vi "GageMultipleRecord_mod_seg.vi"() -> ()   [LabVIEW 2017]
uses:
  <instrlib>/niHWS/nihws.llb/niHWS Open File Permissions ID.ctl
  <instrlib>/niHWS/nihws.llb/niHWS Set Wfm DBL Attribute ID.ctl
  <instrlib>/niHWS/nihws.llb/niHWS Set Wfm DBL Attribute.vi
  <instrlib>/niHWS/nihws.llb/niHWS Write Analog I16.vi
panel:
  out "Numeric":i32
  in  "Number Of Records 2":u32=100
  in  "Save HWS to:":path=path "C:/Users/plasma/Desktop/test.hws"
  out "Segment":u32=1 max=10000
  out "Board":string
  in  "Number Of Records":u32=100
  out "1st segment TS":string
  out "Time Interval Graph":cluster{i32[], dbl[]}(graph)
  out "Tick Frequency, Hz":u32
  in  "Run":bool=TRUE
  in  "Trigger":T1={"Slope"=0, "Level"=0, "Source"=0, "External Range"=2000, "External Coupling"=0, "External"=FALSE, "Disable"=FALSE, "External Impedance"=1} {"External Impedance" items=["50 Ohm", "HiZ"]; "External Coupling" items=["DC", "AC"]; "External Range" min=2000 max=10000 step=8000; "Slope" items=["Rising", "Falling"]; "Level" min=-100 max=100; "Source" min=0 max=64 step=1}
  in  "Reset":bool
  in  "Counter source":bool
  out "Array":dbl[](array[numeric]) format="%.2f"
  out "Status":string
  in  "Channels":T2(array[cluster])=[{"Coupling"=0, "Differential Input"=FALSE, "Direct-to-ADC"=FALSE, "Range"=2000, "Impedance"=50, "DC Offset"=0, "Filter"=0}] {"Impedance" min=50 max=1000000 step=999950; "Coupling" items=["DC", "AC"]}
  in  "Acquisition":T3={"Sample Rate"=10000000.0, "Mode"=0, "Depth"=8160.0, "Segment Size"=8160.0, "Trigger Timeout"=1000000.0, "Trigger Holdoff"=0.0, "Trigger Delay"=0.0, "Clock mode"=enum."Internal"} {"Segment Size" min=32.0 step=16.0; "Trigger Delay" min=0.0 step=1.0; "Trigger Holdoff" min=0.0 step=16.0; "Depth" min=0.0 step=16.0; "Mode" items=["Single", "Dual", "Quad", "Octal"]}
  in  "Stop":bool
  in  "Length":dbl=512.0 min=0.0 step=1.0
  in  "Start Point":dbl step=16.0
  out "Waveform Graph":T4(graph) caption="Record 10000  of  10000"
  # "Time stamp"
  # "of"
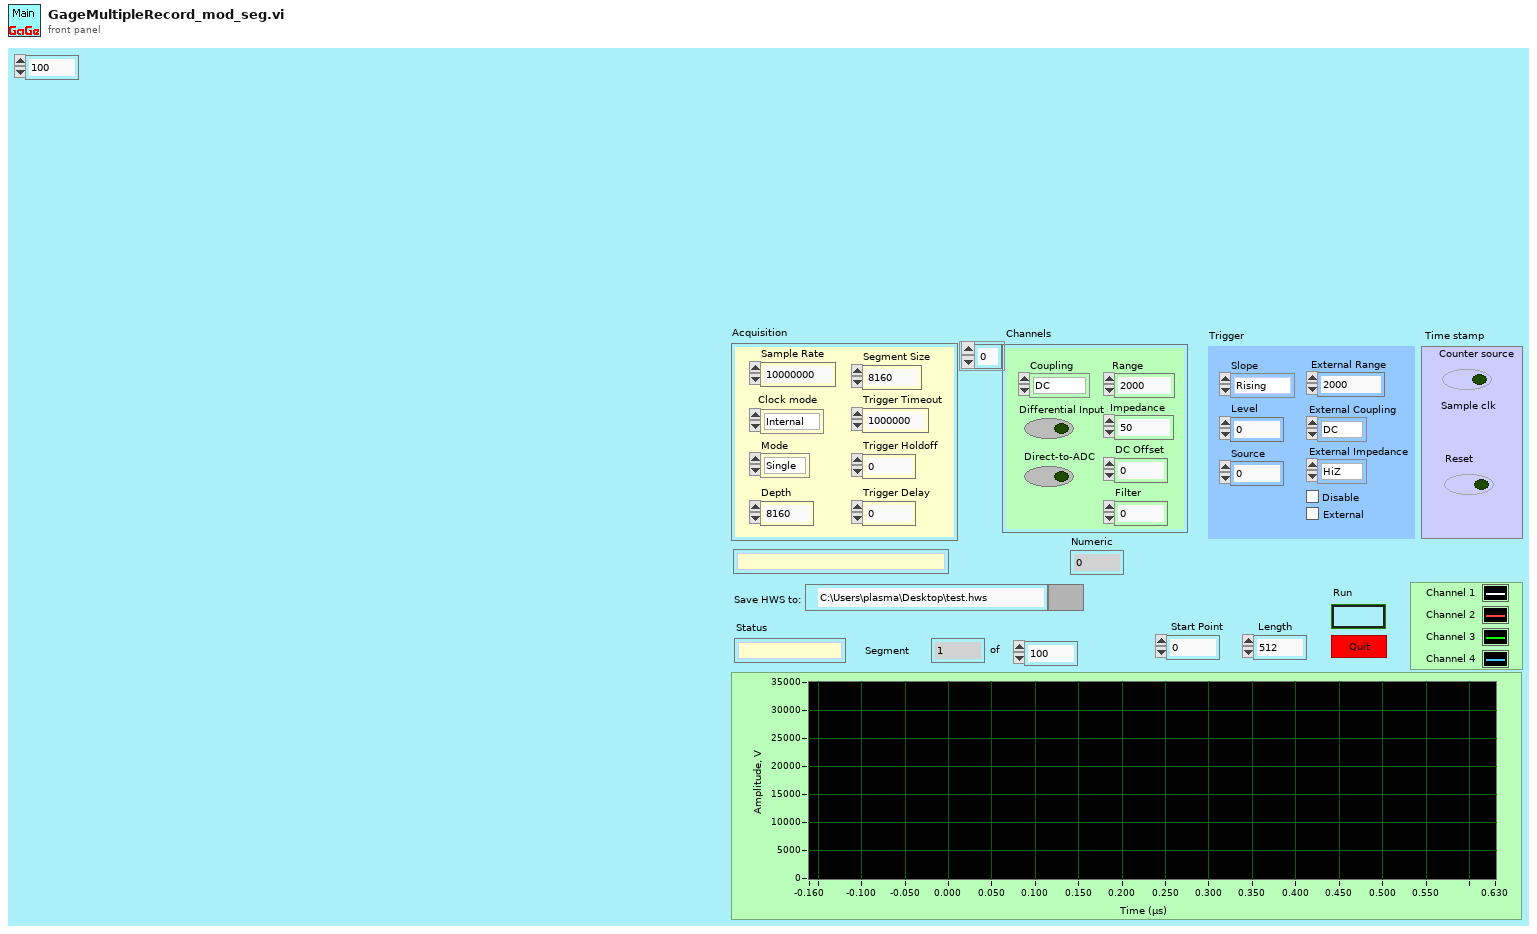
[diagram p1: front panel]
types:
  T1 = cluster{"Slope":u16, "Level":i32, "Source":i32, "External Range":u32, "External Coupling":u16, "External":bool, "Disable":bool, "External Impedance":u16}
  T2 = cluster{"Coupling":u16, "Differential Input":bool, "Direct-to-ADC":bool, "Range":u32, "Impedance":u32, "DC Offset":i32, "Filter":i32}[]
  T3 = cluster{"Sample Rate":dbl, "Mode":u16, "Depth":dbl, "Segment Size":dbl, "Trigger Timeout":dbl, "Trigger Holdoff":dbl, "Trigger Delay":dbl, "Clock mode":enum16{"Internal", "External", "Reference"}}
  T4 = cluster{dbl, dbl, "Data before\n conversion":i16[]}
  T5 = typedef "niHWS Open File Permissions ID.ctl" = enum32{"Read Only", "Read/Write Existing", "Read/Write/Create New", "Read/Write/Create New Always"}
  T6 = cluster{"Handle":u32, "Sample size":u32, "Resolution":i32, "Offset":i32, "Channels":u32, "Boards":u32}
  T7 = cluster{"Coupling":u16, "Differential Input":bool, "Direct-to-ADC":bool, "Range":u32, "Impedance":u32, "DC Offset":i32, "Filter":i32}
  T8 = cluster{string, "Differential Input":bool, "Direct-to-ADC":bool, "Range":u32, "Impedance":u32, "DC Offset":i32, u32}
  T9 = cluster{"RingText.Text":string, "Level":i32, "Source":i32, "External Range":u32, "RingText.Text":string, "External":bool, "Disable":bool, "RingText.Text":string}
  T10 = cluster{"RingText.Text":string, "Level":i32, "Source":i32, "External Range":u32, "RingText.Text":string, "External":bool, "Disable":bool, "RingText.Text":string}[]
  T11 = cluster{"Sample Rate":dbl, "Clock mode":enum16{"Internal", "External", "Reference"}, "RingText.Text":string, "Depth":dbl, "Segment Size":dbl, "Trigger Timeout":dbl, "Trigger Holdoff":dbl, "Trigger Delay":dbl}
  T12 = cluster{"Handle":u32, "Sample Size":u32, "Resolution":i32, "Offset":i32, "Channels":u32, "Boards":u32}
  T13 = typedef "niHWS Set Wfm DBL Attribute ID.ctl" = u32
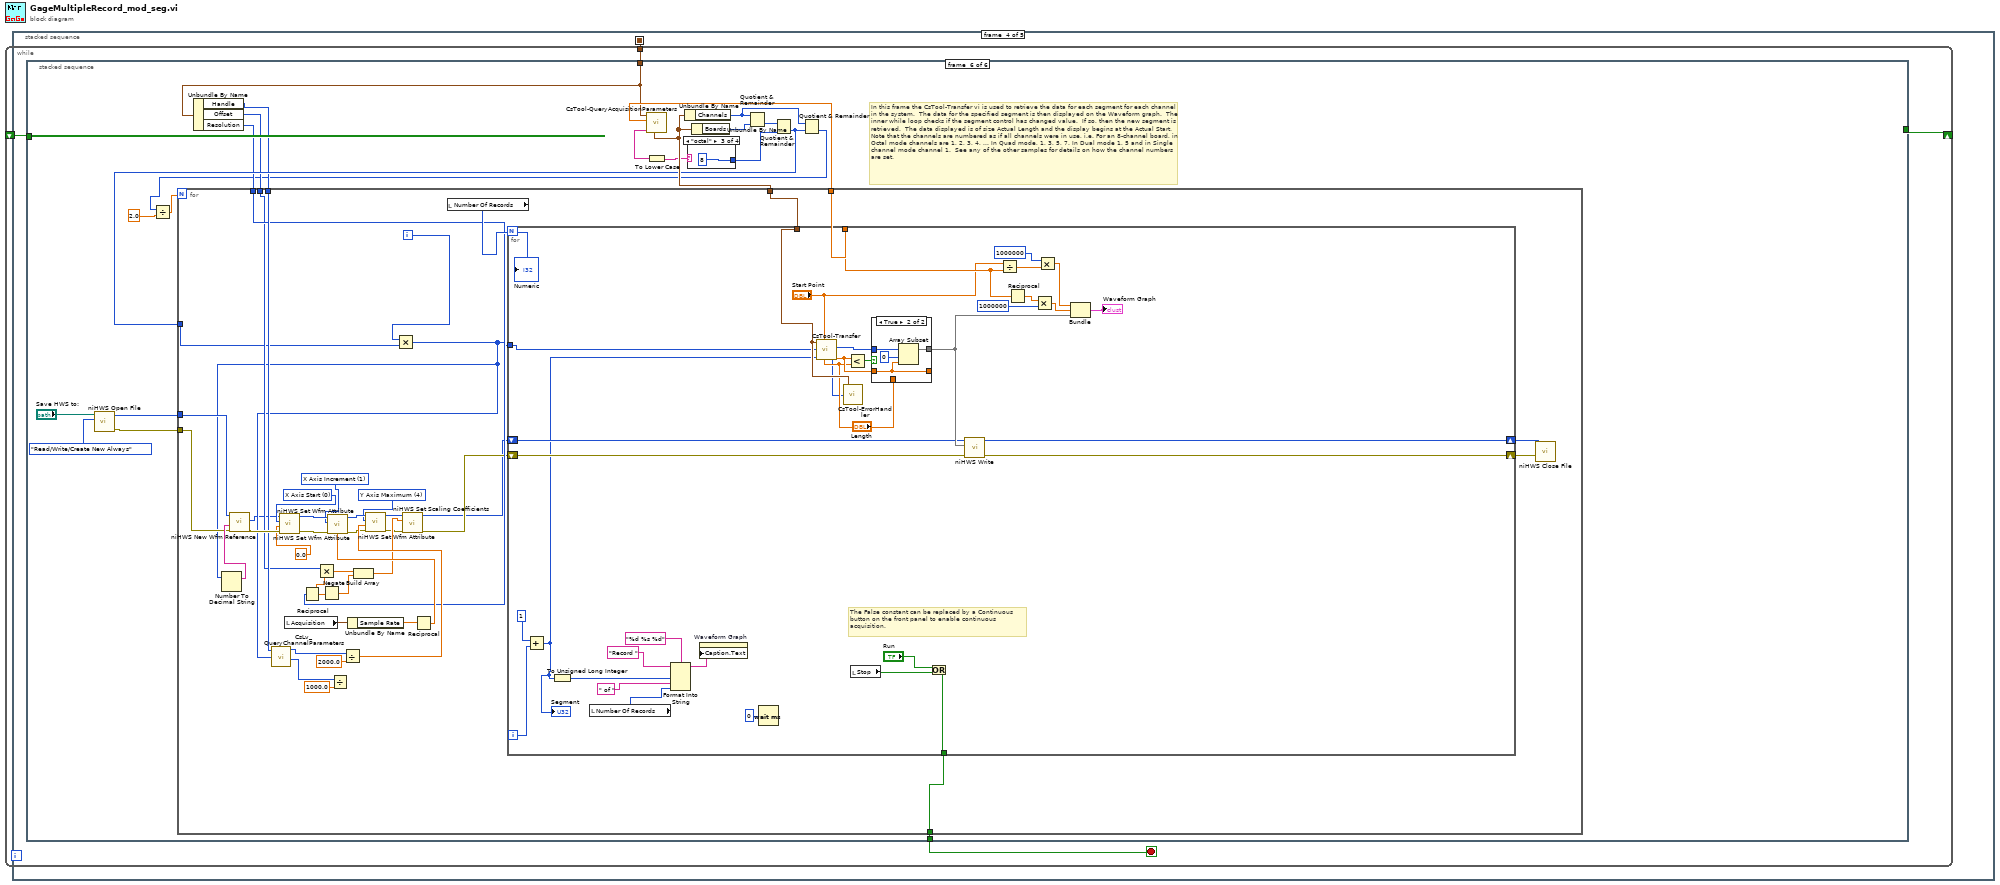
[diagram p0: block diagram]
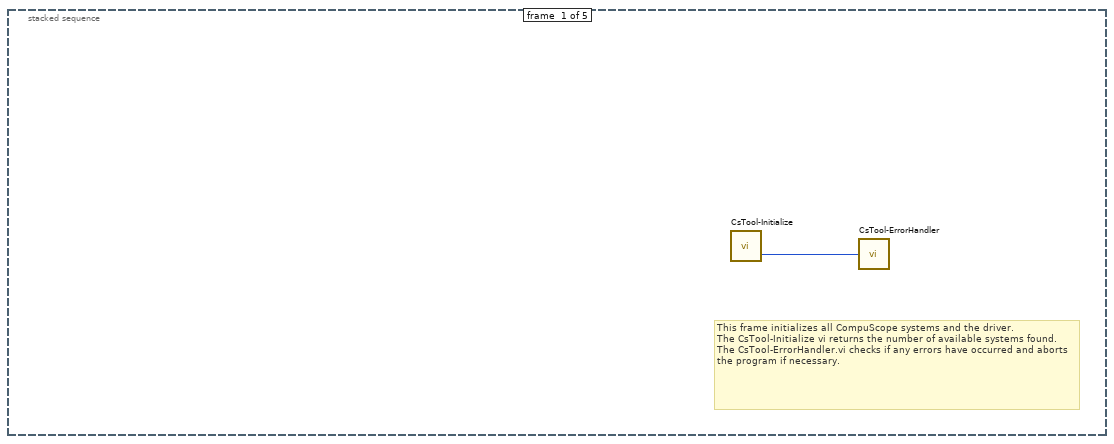
[diagram p2: hidden frame]
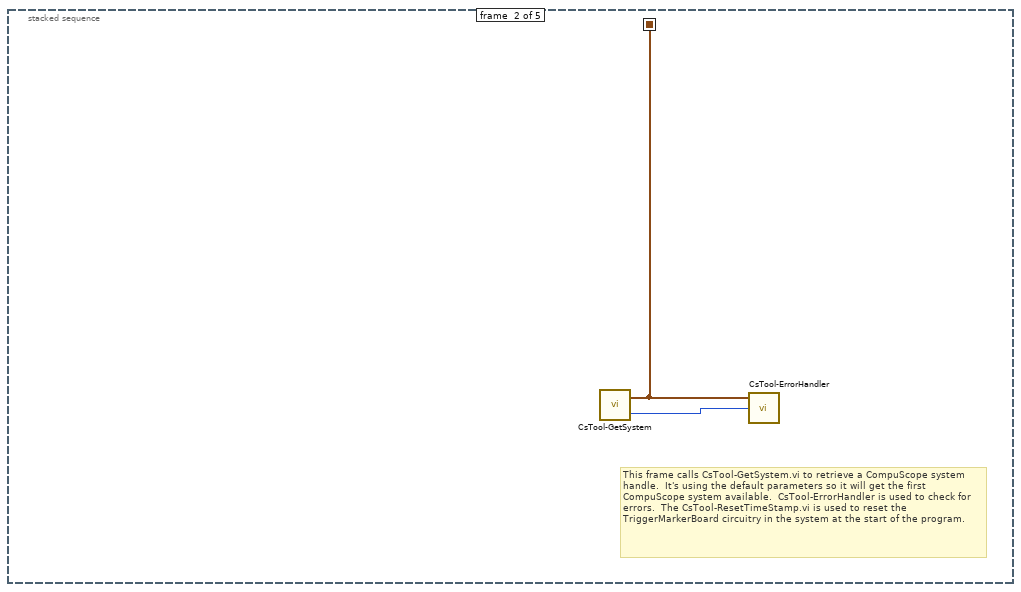
[diagram p3: hidden frame]
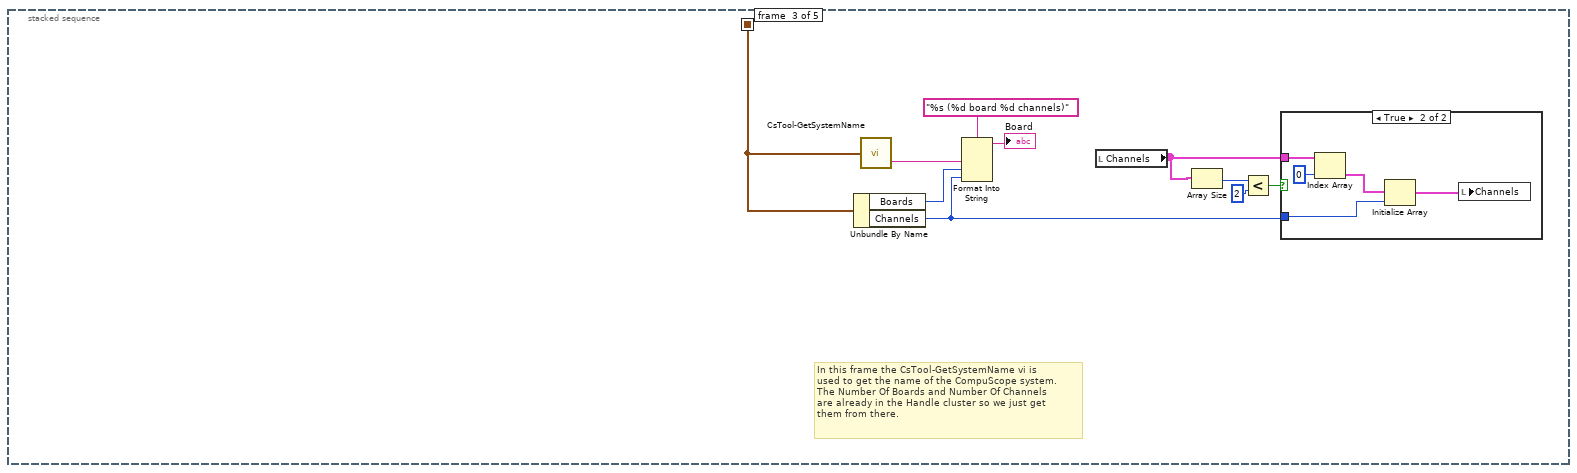
[diagram p4: hidden frame]
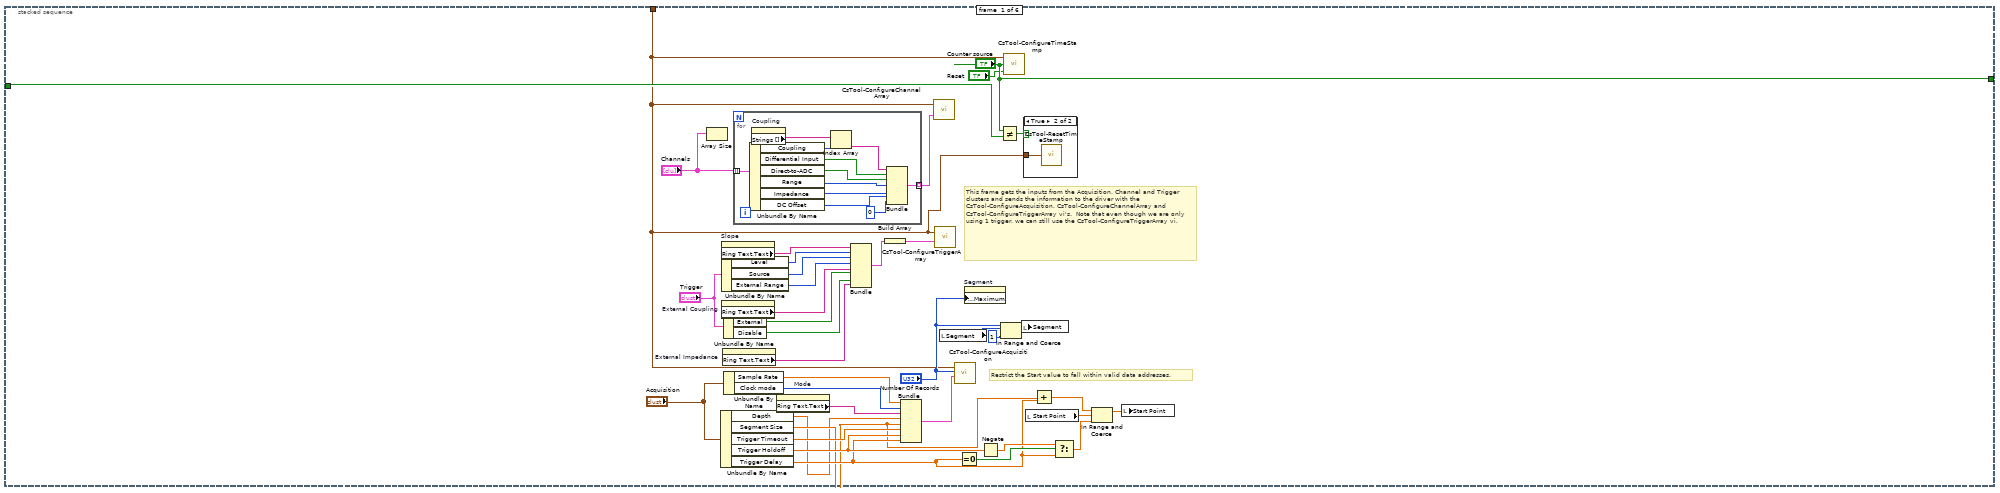
[diagram p6: hidden frame]
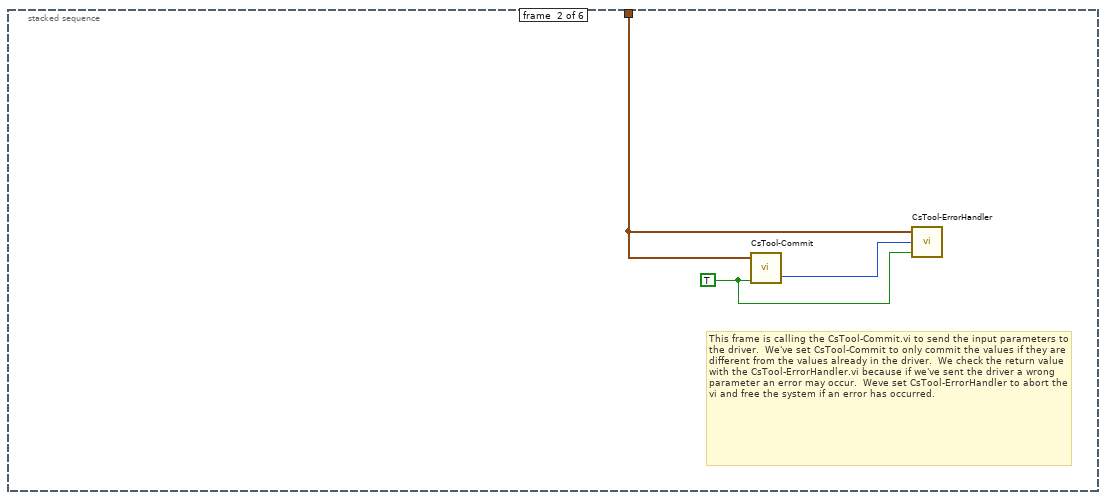
[diagram p8: hidden frame]
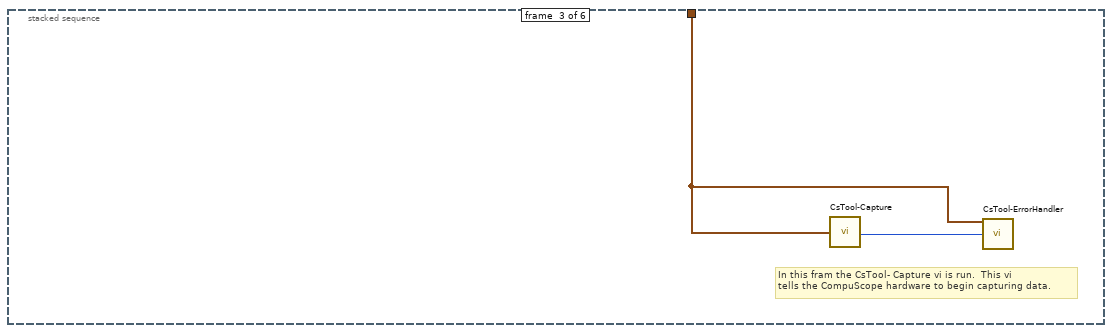
[diagram p9: hidden frame]
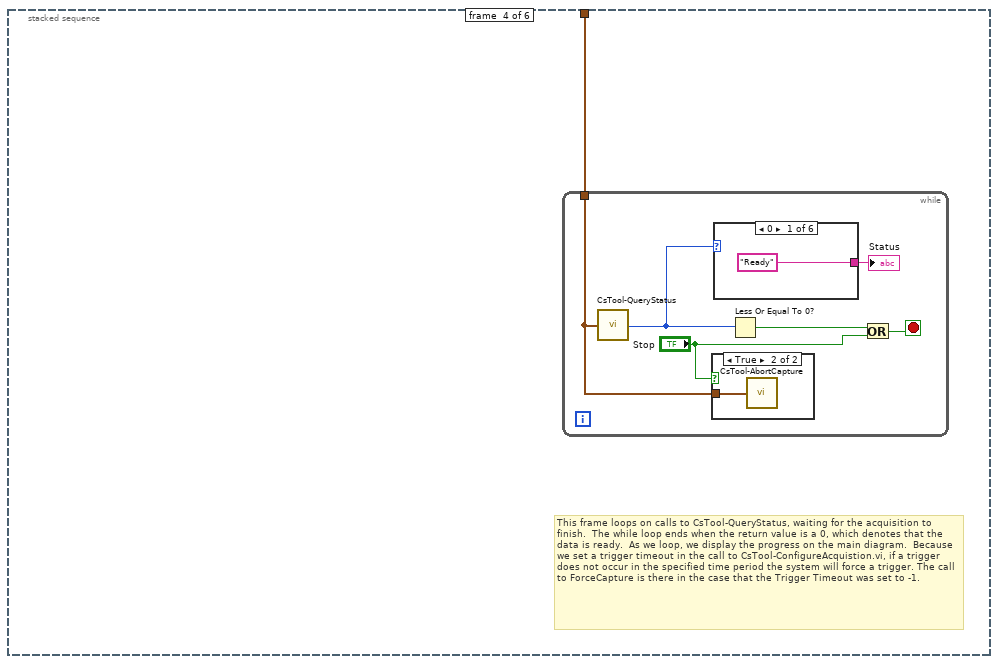
[diagram p10: hidden frame]
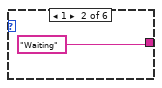
[diagram p12: hidden frame]
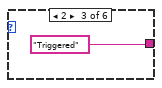
[diagram p13: hidden frame]
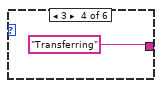
[diagram p14: hidden frame]
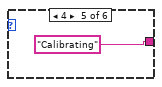
[diagram p15: hidden frame]
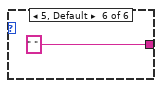
[diagram p16: hidden frame]
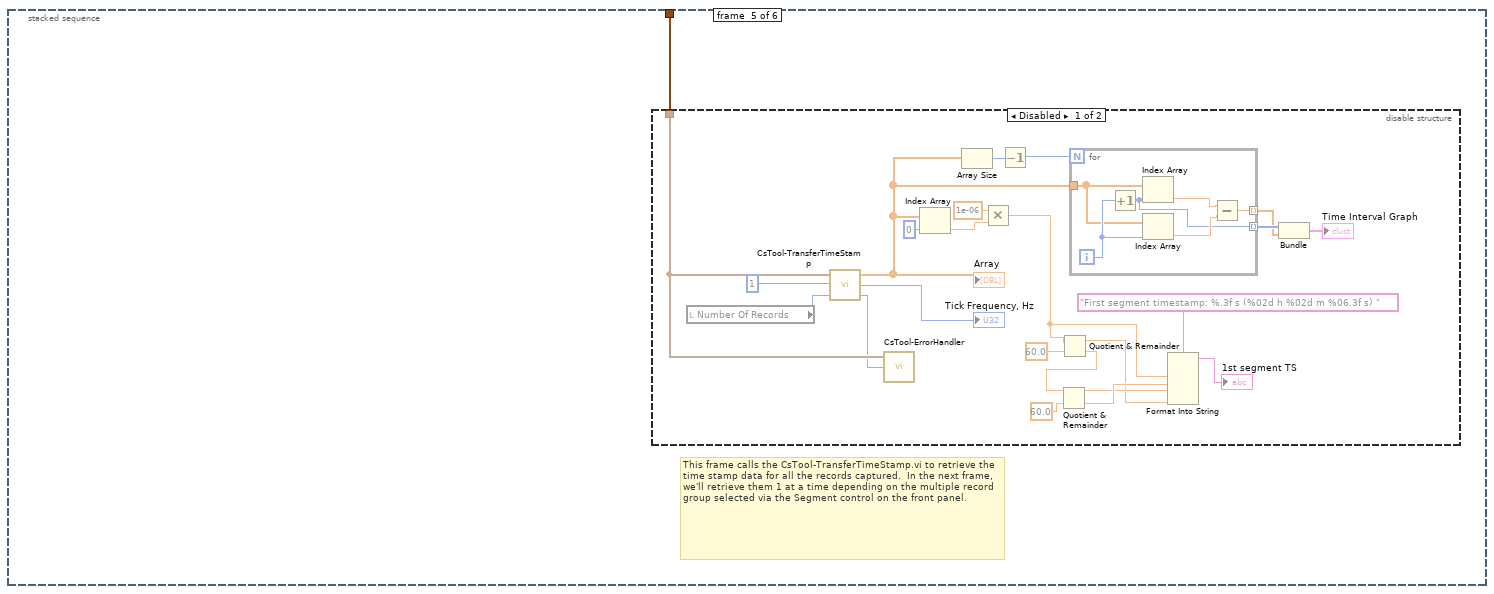
[diagram p17: hidden frame]
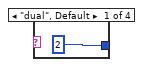
[diagram p20: hidden frame]
diagram:
  n1 = stacked-sequence {
    seq-local: [_ w2 _ _ _] -> [_ _ w13 w19 w231]
    frame #0 {
      # "This frame initializes all CompuScope systems and the driver.\nThe CsTool-Initialize vi returns the number of available systems found.  The CsTool-ErrorHandler.vi checks if any errors have occurred and aborts the program if necessary."
      n2 = call <userlib>:"CsTool-Initialize.vi"() -> ("Error Code"=w1:i32)  [unwired: 1 out]
      n3 = call <userlib>:"CsTool-ErrorHandler.vi"("Error Code"=w1) -> ()  [unwired: 2 in, 1 out]
    }
    frame #1 {
      # "This frame calls CsTool-GetSystem.vi to retrieve a CompuScope system handle.  It's using the default parameters so it will get the first CompuScope system available.  CsTool-ErrorHandler is used to check for errors.  The CsTool-ResetTimeStamp.vi is used to reset the TriggerMarkerBoard circuitry in the system at the start of the program."
      n4 = call <userlib>:"CsTool-GetSystem.vi"() -> ("Error Code"=w3:i32, "Handle Cluster"=w2:T6)  [unwired: 4 in]
      n5 = call <userlib>:"CsTool-ErrorHandler.vi"("Error Code"=w3, "Handle Cluster"=w2) -> ()  [unwired: 1 in, 1 out]
    }
    frame #2 {
      # "In this frame the CsTool-GetSystemName vi is \nused to get the name of the CompuScope system.\nThe Number Of Boards and Number Of Channels \nare already in the Handle cluster so we just get \nthem from there."
      n6 = Unbundle By Name(w13) -> ("Boards"=w5:u32, "Channels"=w6:u32)
      n7 = call <userlib>:"CsTool-GetSystemName.vi"("Handle Cluster"=w13) -> ("System Name"=w7:string)  [unwired: 1 out]
      n8 = Format Into String(format string="%s (%d board %d channels)", w7, w5, w6) -> (resulting string=→"Board":string)  [unwired: 2 in, 1 out]
      n9 = local read "Channels"() -> (w11:T2)
      n10 = Array Size(array=w11) -> (size(s)=w10:i32)
      n11 = Less?(x=w10, y=2) -> (x < y?=w12:bool)
      n12 = case shown="True" w12 {
        tunnel: w6 -> [_ w18]
        tunnel: w11 -> [_ w16]
        frame False {
        }
        frame True {
          n13 = Index Array(array=w16, index=0) -> (element=w15:T7)
          n14 = Initialize Array(w15, w18) -> (w14:T2)
          n15 = local write "Channels"(w14) -> ()
        }
      }
    }
    frame #3 {
      n16 = while {
        tunnel: w19 -> [w23]
        shift-right: [w22] -> _
        shift-left: _ -> [w21]
        stop <- w20 stop-if-true
        n17 = stacked-sequence {
          tunnel: w23 -> [w34 w74 w77 w79 w93 w132]
          tunnel: ["Counter source" _ _ _ _ _] -> w22
          tunnel: w21 -> [w37 _ _ _ _ _]
          tunnel: [_ _ _ _ _ w128] -> w20
          frame #0 {
            # "Restrict the Start value to fall within valid data addresses."
            # "This frame gets the inputs from the Acquisition, Channel and Trigger clusters and sends the information to the driver with the CsTool-ConfigureAcquisition, CsTool-ConfigureChannelArray and CsTool-ConfigureTriggerArray vi's.  Note that even though we are only using 1 trigger, we can still use the CsTool-ConfigureTriggerArray vi."
            n18 = Array Size(array="Channels") -> ()  [unwired: 1 out]
            n19 = Unbundle By Name("Acquisition") -> ("Depth"=w24:dbl, "Segment Size"=w25:dbl, "Trigger Timeout"=w59:dbl, "Trigger Holdoff"=w32:dbl, "Trigger Delay"=w28:dbl)
            n20 = property on="Slope" class="Ring (strict)"() -> ("Ring Text.Text"=w48:string)  [unwired: 2 in, 2 out]
            n21 = Unbundle By Name("Trigger") -> ("Level"=w50:i32, "Source"=w52:i32, "External Range"=w53:u32)
            n22 = property on="External Coupling" class="Ring (strict)"() -> ("Ring Text.Text"=w47:string)  [unwired: 2 in, 2 out]
            n23 = property on="External Impedance" class="Ring (strict)"() -> ("Ring Text.Text"=w46:string)  [unwired: 2 in, 2 out]
            n24 = Unbundle By Name("Trigger") -> ("External"=w51:bool, "Disable"=w54:bool)
            n25 = Unbundle By Name("Acquisition") -> ("Sample Rate"=w57:dbl, "Clock mode"=w58:enum16{"Internal", "External", "Reference"})
            n26 = for {
              tunnel: "Channels" -> [w71] mode=indexing
              tunnel: [w72] -> w60 mode=indexing
              n27 = Unbundle By Name(w71) -> ("Coupling"=w67:u16, "Differential Input"=w73:bool, "Direct-to-ADC"=w66:bool, "Range"=w65:u32, "Impedance"=w64:u32, "DC Offset"=w63:i32)
              n28 = property on="Coupling" class="Ring (strict)"() -> ("Strings []"=w70:string[])  [unwired: 2 in, 2 out]
              n29 = Index Array(array=w70, index=w67) -> (element=w69:string)
              n30 = Bundle(w69, "Differential Input"=w73, "Direct-to-ADC"=w66, "Range"=w65, "Impedance"=w64, "DC Offset"=w63, u32 0) -> (w72:T8)  [unwired: 1 in]
            }
            n31 = property on="Mode" class="Ring (strict)"() -> ("Ring Text.Text"=w56:string)  [unwired: 2 in, 2 out]
            n32 = Bundle("RingText.Text"=w48, "Level"=w50, "Source"=w52, "External Range"=w53, "RingText.Text"=w47, "External"=w51, "Disable"=w54, "RingText.Text"=w46) -> (w45:T9)  [unwired: 1 in]
            n33 = Build Array(w45) -> (w44:T10)
            n34 = Bundle("Sample Rate"=w57, "Clock mode"=w58, "RingText.Text"=w56, "Depth"=w24, "Segment Size"=w25, "Trigger Timeout"=w59, "Trigger Holdoff"=w32, "Trigger Delay"=w28) -> (w43:T11)  [unwired: 1 in]
            n35 = call <userlib>:"CsTool-ConfigureChannelArray.vi"("Channels"=w60, "Handle Cluster"=w34) -> ()  [unwired: 1 out]
            n36 = call <userlib>:"CsTool-ConfigureTriggerArray.vi"("Triggers"=w44, "Handle Cluster"=w34) -> ()  [unwired: 1 out]
            n37 = local read "Segment"() -> (w39:u32)
            n38 = call <userlib>:"CsTool-ConfigureAcquisition.vi"("Handle Cluster"=w34, "Segment Count (1)"="Number Of Records", "Acquisition"=w43) -> ()  [unwired: 2 in, 1 out]
            n39 = Equal To 0?(x=w28) -> (x = 0?=w31:bool)
            n40 = property on="Segment" class="DigNum (strict)"("Data Entry Limits:Maximum"="Number Of Records") -> ()  [unwired: 2 in, 2 out]
            n41 = Negate(x=w32) -> (-x=w30:dbl)
            n42 = Not Equal?(x="Counter source", y=w37) -> (x != y?=w38:bool)
            n43 = In Range and Coerce(upper limit="Number Of Records", x=w39, lower limit=u32 1) -> (coerced(x)=w42:u32)  [unwired: 1 out]
            n44 = call <userlib>:"CsTool-ConfigureTimeStamp.vi"("Reset"="Reset", "Sample Clock"="Counter source", "Handle Cluster"=w34) -> ()  [unwired: 1 out]
            n45 = local write "Segment"(w42) -> ()
            n46 = case shown="True" w38 {
              tunnel: w34 -> [_ w62]
              frame False {
              }
              frame True {
                n47 = call <userlib>:"CsTool-ResetTimeStamp.vi"("Handle Cluster"=w62) -> ()  [unwired: 1 out]
              }
            }
            n48 = local read "Start Point"() -> (w33:dbl)
            n49 = Add(x=w25, y=w28) -> (x+y=w27:dbl)
            n50 = Select(t=w30, s=w31, f=w28) -> (s? t:f=w29:dbl)
            n51 = In Range and Coerce(upper limit=w27, x=w33, lower limit=w29) -> (coerced(x)=w26:dbl)  [unwired: 1 out]
            n52 = local write "Start Point"(w26) -> ()
          }
          frame #1 {
            w75 = TRUE
            # "This frame is calling the CsTool-Commit.vi to send the input parameters to the driver.  We've set CsTool-Commit to only commit the values if they are different from the values already in the driver.  We check the return value with the CsTool-ErrorHandler.vi because if we've sent the driver a wrong parameter an error may occur.  Weve set CsTool-ErrorHandler to abort the vi and free the system if an error has occurred."
            n53 = call <userlib>:"CsTool-Commit.vi"("OnlyOnChange (t)"=w75, "Handle Cluster"=w74) -> ("Error Code"=w76:i32)  [unwired: 1 in, 1 out]
            n54 = call <userlib>:"CsTool-ErrorHandler.vi"("StopOnError (true)"=w75, "Error Code"=w76, "Handle Cluster"=w74) -> ()  [unwired: 1 out]
          }
          frame #2 {
            # "In this fram the CsTool- Capture vi is run.  This vi\ntells the CompuScope hardware to begin capturing data."
            n55 = call <userlib>:"CsTool-Capture.vi"("Handle Cluster"=w77) -> ("Error Code"=w78:i32)
            n56 = call <userlib>:"CsTool-ErrorHandler.vi"("Error Code"=w78, "Handle Cluster"=w77) -> ()  [unwired: 1 in, 1 out]
          }
          frame #3 {
            # "This frame loops on calls to CsTool-QueryStatus, waiting for the acquisition to finish.  The while loop ends when the return value is a 0, which denotes that the data is ready.  As we loop, we display the progress on the main diagram.  Because we set a trigger timeout in the call to CsTool-ConfigureAcquistion.vi, if a trigger does not occur in the specified time period the system will force a trigger. The call to ForceCapture is there in the case that the Trigger Timeout was set to -1."
            n57 = while {
              tunnel: w79 -> [w81]
              stop <- w83 stop-if-true
              n58 = call <userlib>:"CsTool-QueryStatus.vi"("Handle Cluster"=w81) -> ("Status"=w82:i32)
              n59 = case shown="True" "Stop" {
                tunnel: w81 -> [_ w86]
                frame False {
                }
                frame True {
                  n60 = call <userlib>:"CsTool-AbortCapture.vi"("Handle Cluster"=w86) -> ()  [unwired: 1 out]
                }
              }
              n61 = case shown="0" w82 {
                tunnel: ["Ready" "Waiting" "Triggered" "Transferring" "Calibrating" " "] -> w85
                frame 0 {
                }
                frame 1 {
                }
                frame 2 {
                }
                frame 3 {
                }
                frame 4 {
                }
                frame 5, Default {
                }
              }
              "Status" <- w85
              n62 = Less Or Equal To 0?(x=w82) -> (x <= 0?=w84:bool)
              n63 = Or(x=w84, y="Stop") -> (x .or. y?=w83:bool)
            }
          }
          frame #4 {
            # "This frame calls the CsTool-TransferTimeStamp.vi to retrieve the time stamp data for all the records captured.  In the next frame, we'll retrieve them 1 at a time depending on the multiple record group selected via the Segment control on the front panel."
            n64 = disable-structure shown="Disabled" {
              disable-tunnel: w93 -> [w95 _]
              frame Disabled {
                n65 = local read "Number Of Records"() -> (w115:u32)
                n66 = call <userlib>:"CsTool-TransferTimeStamp.vi"("Length (1)"=w115, "Segment (1)"=1, "Handle Cluster"=w95) -> ("Error Code"=w94:i32, "Tick Frequency"=→"Tick Frequency, Hz":u32, "TS Time"=w111:dbl[])
                "Array" <- w111
                n67 = call <userlib>:"CsTool-ErrorHandler.vi"("Error Code"=w94, "Handle Cluster"=w95) -> ()  [unwired: 1 in, 1 out]
                n68 = Index Array(array=w111, index=0) -> (element=w109:dbl)
                n69 = Array Size(array=w111) -> (size(s)=w113:i32)
                n70 = Multiply(x=1e-06, y=w109) -> (x*y=w103:dbl)
                n71 = Decrement(x=w113) -> (x-1=w112:i32)
                n72 = Quotient & Remainder(x=w103, y=60.0) -> (x-y*floor(x/y)=w100:dbl, floor(x/y)=w106:dbl)
                n73 = Quotient & Remainder(x=w106, y=60.0) -> (x-y*floor(x/y)=w101:dbl, floor(x/y)=w102:dbl)
                n74 = for {
                  N: w112 -> [_]
                  tunnel: w111 -> [w119]
                  tunnel: [w118] -> w97 mode=indexing
                  tunnel: [w117] -> w98 mode=indexing
                  i -> [w122]
                  n75 = Increment(x=w122) -> (x+1=w117:i32)
                  n76 = Index Array(array=w119, index=w117) -> (element=w121:dbl)
                  n77 = Index Array(array=w119, index=w122) -> (element=w120:dbl)
                  n78 = Subtract(x=w121, y=w120) -> (x-y=w118:dbl)
                }
                n79 = Format Into String(format string="First segment timestamp: %.3f s (%02d h %02d m %06.3f s) ", w103, w102, w101, w100) -> (resulting string=→"1st segment TS":string)  [unwired: 2 in, 1 out]
                n80 = Bundle(w98, w97) -> (→"Time Interval Graph":cluster{i32[], dbl[]})  [unwired: 1 in]
              }
              frame Enabled {
              }
            }
          }
          frame #5 {
            # "In this frame the CsTool-Transfer vi is used to retrieve the data for each segment for each channel in the system.  The data for the specified segment is then displayed on the Waveform graph.  The inner while loop checks if the segment control has changed value.  If so, then the new segment is retrieved.  The data displayed is of size Actual Length and the display begins at the Actual Start. Note that the channels are numbered as if all channels were in use, i.e. For an 8-channel board, in Octal mode channels are 1, 2, 3, 4, ... In Quad mode, 1, 3, 5, 7. In Dual mode 1, 5 and in Single channel mode channel 1.  See any of the other samples for details on how the channel numbers are set."
            n81 = call <instrlib>:"niHWS Open File.vi"("permissions (0:read only)"=niHWS_Open_File_Permissions_ID."Read/Write/Create New Always", "file path"="Save HWS to:") -> ("error out"=w126:errorcluster, "file handle"=w127:u32)  [unwired: 8 in]
            n82 = Unbundle By Name(w132) -> ("Handle"=w130:u32, "Offset"=w131:i32, "Resolution"=w129:i32)
            n83 = call <userlib>:"CsTool-QueryAcquisitionParameters.vi"("Handle Cluster"=w132) -> ("Output Handle Cluster"=w142:T12, "Mode"=w141:string, "Sample Rate"=w143:dbl)  [unwired: 8 out]
            n84 = To Lower Case(string=w141) -> (all lower case string=w140:string)
            n85 = Unbundle By Name(w142) -> ("Channels"=w136:u32)
            n86 = case shown="\"octal\"" w140 {
              tunnel: [2 4 8 1] -> w137
              frame "dual", Default {
              }
              frame "quad" {
              }
              frame "octal" {
              }
              frame "single" {
              }
            }
            n87 = Unbundle By Name(w142) -> ("Boards"=w139:u32)
            n88 = Quotient & Remainder(x=w136, y=w139) -> (floor(x/y)=w138:u32)  [unwired: 1 out]
            n89 = Quotient & Remainder(x=w138, y=w137) -> (floor(x/y)=w135:u32)  [unwired: 1 out]
            n90 = Quotient & Remainder(x=w136, y=w135) -> (floor(x/y)=w124:u32)  [unwired: 1 out]
            n91 = Divide(x=w124, y=2.0) -> (x/y=w123:dbl)
            n92 = for {
              N: w123 -> [_]
              tunnel: w143 -> [w184]
              tunnel: w142 -> [w183]
              tunnel: w135 -> [w144]
              tunnel: w131 -> [w155]
              tunnel: w130 -> [w159]
              tunnel: w129 -> [w156]
              tunnel: [w182] -> w128
              tunnel: w127 -> [w157]
              tunnel: w126 -> [w158]
              i -> [w181]
              w153 = T13 0 items=["X Axis Start"=0, "X Axis Increment"=1, "Y Axis Minimum"=3, "Y Axis Maximum"=4] ("attribute ID")
              w152 = T13 1 items=["X Axis Start"=0, "X Axis Increment"=1, "Y Axis Minimum"=3, "Y Axis Maximum"=4] ("attribute ID")
              w151 = T13 4 items=["X Axis Start"=0, "X Axis Increment"=1, "Y Axis Minimum"=3, "Y Axis Maximum"=4] ("attribute ID")
              n93 = local read "Acquisition"() -> (w173:T3)
              n94 = Reciprocal(x=w156) -> (1/x=w170:dbl)
              n95 = Multiply(x=w155, y=w170) -> (x*y=w169:dbl)
              n96 = Negate(x=w170) -> (-x=w171:dbl)
              n97 = Unbundle By Name(w173) -> ("Sample Rate"=w174:dbl)
              n98 = Build Array(w169, w171) -> (w168:dbl[])
              n99 = Multiply(x=w181, y=w144) -> (x*y=w148:u32)
              n100 = Number To Decimal String(number=w148) -> (decimal integer string=w178:string)  [unwired: 1 in]
              n101 = call <instrlib>:"niHWS New Wfm Reference.vi"("error in (no error)"=w158, "waveform name (empty)"=w178, "file handle in"=w157) -> ("error out"=w179:errorcluster, "waveform reference"=w145:u32)  [unwired: 6 in, 1 out]
              n102 = call <userlib>:"CsLv_QueryChannelParameters.vi"("Channel"=w148, "Handle"=w159) -> ("DC Offset (mV)"=w176:i32, "Input Range (mV)"=w175:u32)  [unwired: 5 out]
              n103 = call-poly <instrlib>:"niHWS Set Wfm Attribute.vi"("error in (no error)"=w179, "attribute value"=0.0, "attribute ID"=w153, "waveform reference in"=w145) -> ("error out"=w166:errorcluster, "waveform reference out"=w167:u32)  [unwired: 6 in]
              n104 = Divide(x=w176, y=1000.0) -> ()  [unwired: 1 out]
              n105 = Divide(x=w175, y=2000.0) -> (x/y=w177:dbl)
              n106 = Reciprocal(x=w174) -> (1/x=w172:dbl)
              n107 = call-poly <instrlib>:"niHWS Set Wfm Attribute.vi"("error in (no error)"=w166, "attribute value"=w172, "attribute ID"=w152, "waveform reference in"=w167) -> ("error out"=w165:errorcluster, "waveform reference out"=w163:u32)  [unwired: 6 in]
              n108 = call-poly <instrlib>:"niHWS Set Wfm Attribute.vi"("error in (no error)"=w165, "attribute value"=w177, "attribute ID"=w151, "waveform reference in"=w163) -> ("error out"=w164:errorcluster, "waveform reference out"=w162:u32)  [unwired: 6 in]
              n109 = call <instrlib>:"niHWS Set Scaling Coefficients.vi"("error in (no error)"=w164, "coefficient array"=w168, "waveform reference in"=w162) -> ("error out"=w150:errorcluster, "waveform reference out"=w149:u32)  [unwired: 7 in]
              n110 = local read "Number Of Records"() -> (w180:u32)
              n111 = for {
                N: w180 -> [w192]
                tunnel: w184 -> [w219]
                tunnel: w183 -> [w218]
                tunnel: [w201] -> w182
                tunnel: w148 -> [w185]
                shift-right: [w193] -> w146
                shift-left: w149 -> [w188]
                shift-right: [w194] -> w147
                shift-left: w150 -> [w189]
                i -> [w191]
                # "The False constant can be replaced by a Continuous\nbutton on the front panel to enable continuous\nacquisition."
                n112 = Add(x=1, y=w191) -> (x+y=w186:i32)
                "Segment" <- w186
                n113 = To Unsigned Long Integer(number=w186) -> (unsigned 32bit integer=w195:u32)
                n114 = local read "Number Of Records"() -> (w200:u32)
                n115 = Format Into String(format string="%d %s %d", initial string="Record ", w195, " of ", w200) -> (resulting string=w199:string)  [unwired: 1 in, 1 out]
                n116 = property on="Waveform Graph" class="WFGraph (strict)"("Caption.Text"=w199) -> ()  [unwired: 2 in, 2 out]
                n117 = Wait (ms)(milliseconds to wait=u32 0) -> ()  [unwired: 1 out]
                n118 = call <userlib>:"CsTool-Transfer.vi"("Length (4096)"="Length", "Start (0)"="Start Point", "Segment (1)"=w186, "Channel (0)"=w185, "Handle Cluster"=w218) -> ("Error Code"=w205:i32, "Actual Length"=w207:dbl, "Data before\n conversion"=w208:i16[])  [unwired: 1 in, 1 out]
                n119 = call <userlib>:"CsTool-ErrorHandler.vi"("Error Code"=w205, "Handle Cluster"=w218) -> ()  [unwired: 1 in, 1 out]
                n120 = Less?(x=w207, y="Length") -> (x < y?=w209:bool)
                n121 = local read "Stop"() -> (w202:bool)
                n122 = case shown="True" w209 {
                  tunnel: w208 -> [w221 w225]
                  tunnel: [w221 w223] -> w204
                  tunnel: w207 -> [_ w222]
                  tunnel: [w220 w222] -> _
                  tunnel: "Length" -> [w220 _]
                  frame False {
                  }
                  frame True {
                    n123 = Array Subset(array=w225, index=0, length=w222) -> (w223:i16[])
                  }
                }
                n124 = Or(x="Run", y=w202) -> (x .or. y?=w201:bool)
                n125 = call-poly <instrlib>:"niHWS Write.vi"("error in (no error)"=w189, "data"=w204, "waveform reference in"=w188) -> ("error out"=w194:errorcluster, "waveform reference out"=w193:u32)  [unwired: 7 in]
                n126 = Divide(x="Start Point", y=w219) -> (x/y=w211:dbl)
                n127 = Reciprocal(x=w219) -> (1/x=w212:dbl)
                n128 = Multiply(x=w212, y=1000000) -> (x*y=w215:dbl)
                n129 = Multiply(x=1000000, y=w211) -> (x*y=w214:dbl)
                n130 = Bundle(w214, w215, "Data before\n conversion"=w204) -> (→"Waveform Graph":T4)  [unwired: 1 in]
                "Numeric" <- w192
              }
              n131 = call <instrlib>:"niHWS Close File.vi"("error in (no error)"=w147, "file handle"=w146) -> ()  [unwired: 9 in, 1 out]
            }
          }
        }
      }
    }
    frame #4 {
      # "We set the Stop button (actually it's local variable) to False here so when the vi stops the Stop button will not stay depressed."
      # "In this frame, which is reached when the Stop\nis pressed, the CompuScope system is freed by\nrunning the CsTool-FreeSystem vi.  This frees any resources\nused by the system and makes it available for another\nprogram to use."
      n132 = local write "Stop"(FALSE) -> ()
      n133 = call <userlib>:"CsTool-FreeSystem.vi"("Handle Cluster"=w231) -> ()  [unwired: 1 out]
    }
  }
